vi "TurretGuide.vi"(4 "Right Stop":bool, 6 "Left Stop":bool, 7 "Angle Not Stale":bool, 8 "error in (no error)":errorcluster, 9 "Angle Margin":dbl, 10 "Angle to Target":dbl, 11 "Image":T1) -> (0 "Drawing Mode (Frame)":u32, 1 "error out":errorcluster, 3 "Image Out":T1)   [LabVIEW 2013]
uses:
  <vilib>/vision/Image Controls.llb/IMAQ Image.ctl
panel:
  # "This VI takes in the Angle to Target and applies the following to the Screen Image\n1) Gives Left or Right arrows directing the Operator to center the Turret on Target\n2) Tell operator when Turrent is centered within a certain margin on Target\n3) Tells Operator when Hardstops have been hit"
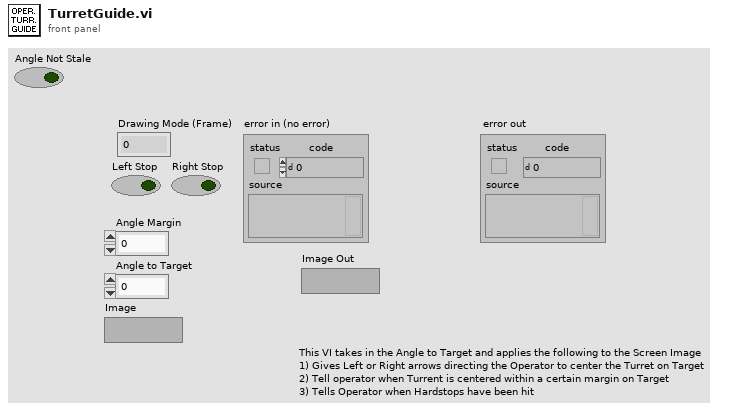
[diagram p1: front panel]
types:
  T1 = typedef "IMAQ Image.ctl" = refnum<image>
  T2 = cluster{"Left":i32, "Top":i32, "Right":i32, "Bottom":i32}
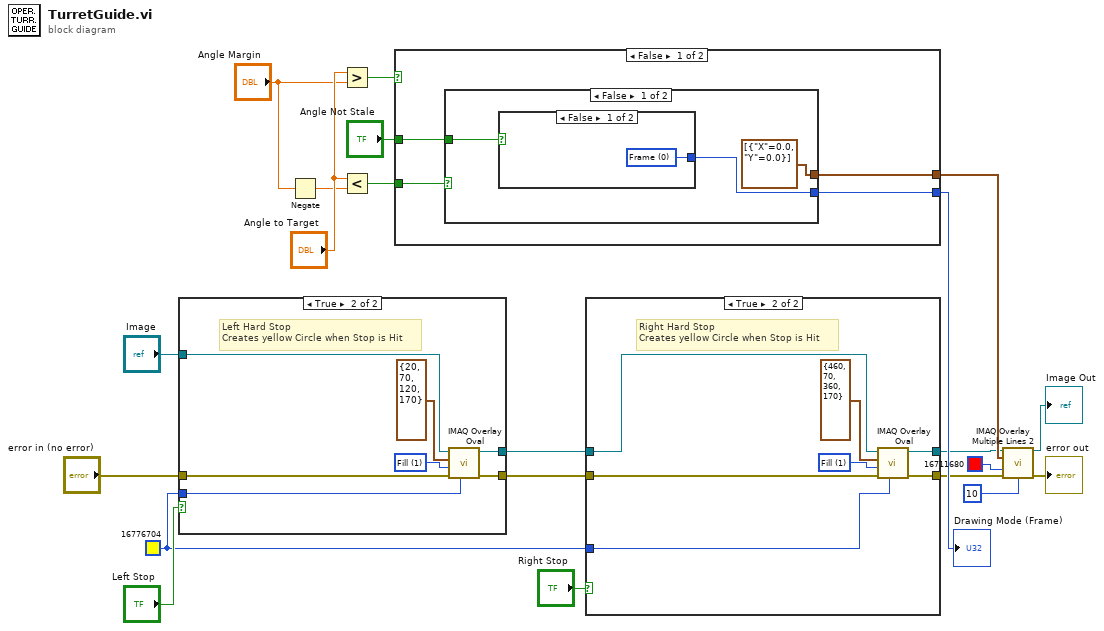
[diagram p0: block diagram]
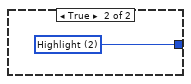
[diagram p4: hidden frame]
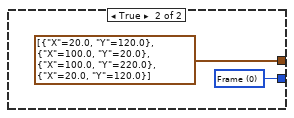
[diagram p5: hidden frame]
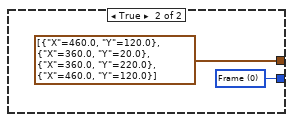
[diagram p6: hidden frame]
diagram:
  w2 = u32 16776704 ("Color")
  n1 = case shown="True" "Left Stop" {
    tunnel: "error in (no error)" -> [w22 w30]
    tunnel: [w22 w29] -> w6
    tunnel: "Image" -> [w23 w28]
    tunnel: [w23 w27] -> w8
    tunnel: w2 -> [_ w24]
    frame False {
    }
    frame True {
      w26 = u32 1 items=["Frame", "Fill"] ("Drawing Mode (Frame)")
      # "Left Hard Stop\nCreates yellow Circle when Stop is Hit"
      n2 = call "IMAQ Overlay Oval"("Color"=w24, "error in (no error)"=w30, "Drawing Mode (Frame)"=w26, "Bounding Rectangle"=T2 {"Left"=20, "Top"=70, "Right"=120, "Bottom"=170}, "Image"=w28) -> ("error out"=w29:errorcluster, "Image Out"=w27:T1)  [unwired: 5 in]
    }
  }
  n3 = Negate(x="Angle Margin") -> (-x=w15:dbl)
  n4 = Greater?(x="Angle to Target", y="Angle Margin") -> (0:w21:bool)
  n5 = Less?(x="Angle to Target", y=w15) -> (x < y?=w20:bool)
  n6 = case shown="False" w21 {
    tunnel: w20 -> [w34 _]
    tunnel: [w33 cluster{"X":dbl, "Y":dbl}[] [{"X"=460.0, "Y"=120.0}, {"X"=360.0, "Y"=20.0}, {"X"=360.0, "Y"=220.0}, {"X"=460.0, "Y"=120.0}] ("Line End Points")] -> w16
    tunnel: [w32 w43] -> w13
    tunnel: "Angle Not Stale" -> [w31 _]
    frame False {
      n7 = case shown="False" w34 {
        tunnel: [cluster{"X":dbl, "Y":dbl}[] [{"X"=0.0, "Y"=0.0}] ("Line End Points") cluster{"X":dbl, "Y":dbl}[] [{"X"=20.0, "Y"=120.0}, {"X"=100.0, "Y"=20.0}, {"X"=100.0, "Y"=220.0}, {"X"=20.0, "Y"=120.0}] ("Line End Points")] -> w33
        tunnel: [w36 w40] -> w32
        tunnel: w31 -> [w35 _]
        frame False {
          n8 = case shown="False" w35 {
            tunnel: [w38 w39] -> w36
            frame False {
              w38 = u32 0 items=["Frame", "Fill", "Highlight"] ("Drawing Mode (Frame)")
            }
            frame True {
              w39 = u32 2 items=["Frame", "Fill", "Highlight"] ("Drawing Mode (Frame)")
            }
          }
        }
        frame True {
          w40 = u32 0 items=["Frame", "Fill", "Highlight"] ("Drawing Mode (Frame)")
        }
      }
    }
    frame True {
      w43 = u32 0 items=["Frame", "Fill", "Highlight"] ("Drawing Mode (Frame)")
    }
  }
  "Drawing Mode (Frame)" <- w13
  n9 = case shown="True" "Right Stop" {
    tunnel: w6 -> [w44 w52]
    tunnel: [w44 w51] -> w5
    tunnel: w8 -> [w45 w50]
    tunnel: [w45 w49] -> w7
    tunnel: w2 -> [_ w46]
    frame False {
    }
    frame True {
      w48 = u32 1 items=["Frame", "Fill"] ("Drawing Mode (Frame)")
      # "Right Hard Stop\nCreates yellow Circle when Stop is Hit"
      n10 = call "IMAQ Overlay Oval"("Color"=w46, "error in (no error)"=w52, "Drawing Mode (Frame)"=w48, "Bounding Rectangle"=T2 {"Left"=460, "Top"=70, "Right"=360, "Bottom"=170}, "Image"=w50) -> ("error out"=w51:errorcluster, "Image Out"=w49:T1)  [unwired: 5 in]
    }
  }
  n11 = call "IMAQ Overlay Multiple Lines 2"("Image"=w7, "Line End Points"=w16, "Color"=u32 16711680, "error in (no error)"=w5, "Width"=u32 10) -> ("Image Out"=→"Image Out":T1, "error out"=→"error out":errorcluster)  [unwired: 9 in]
